vi "Simple TCP - Server.vi"() -> ()   [LabVIEW 2024]
doc: "Demonstrates how to set up a basic TCP connection, send data to the specified port once a connection has been established, and terminate the connection once the data has been sent. This VI is designed to stop if the TCP connection is terminated. The data sent in this example is an array of random numbers."
panel:
  in  "Client Closed":string="The client VI closed the connection."
  out "Waveform Graph":dbl[](graph)
  # "Overview: Demonstrates the use of the TCP functions to initialize a TCP server that can send data to a client VI.\nInstructions:\n1. Run the VI.\n2. Open Simple TCP - Client.vi and follow the instructions on its front panel. Note that if you wait longer than 30 seconds to do this after running this VI, it will time out.\n3. Click Stop on Simple TCP - Client.vi. This VI will stop automatically."
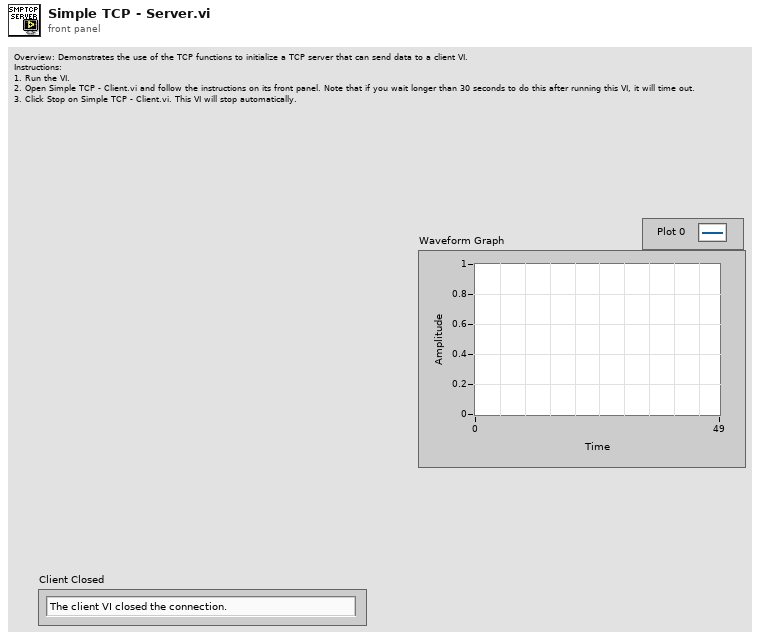
[diagram p1: front panel]
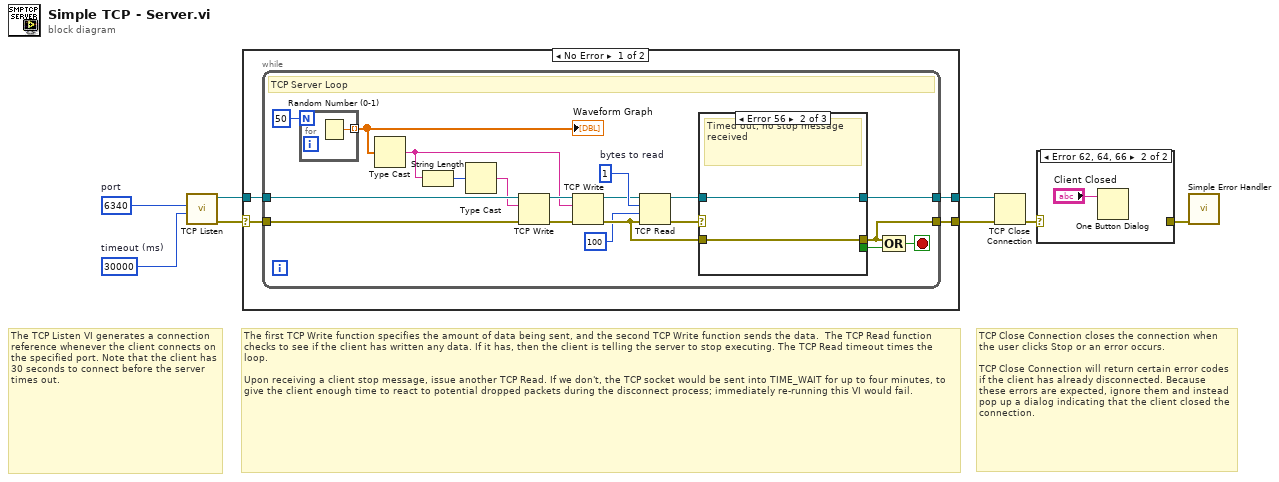
[diagram p0: block diagram]
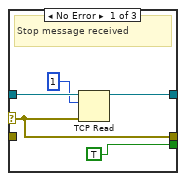
[diagram p2: hidden frame]
diagram:
  w3 = u16 6340  # port
  w4 = 30000  # timeout (ms)
  # "TCP Close Connection closes the connection when the user clicks Stop or an error occurs.\n\nTCP Close Connection will return certain error codes if the client has already disconnected. Because these errors are expected, ignore them and instead pop up a dialog indicating that the client closed the connection."
  # "The TCP Listen VI generates a connection reference whenever the client connects on the specified port. Note that the client has 30 seconds to connect before the server times out."
  # "The first TCP Write function specifies the amount of data being sent, and the second TCP Write function sends the data.  The TCP Read function checks to see if the client has written any data. If it has, then the client is telling the server to stop executing. The TCP Read timeout times the loop.\n\nUpon receiving a client stop message, issue another TCP Read. If we don't, the TCP socket would be sent into TIME_WAIT for up to four minutes, to give the client enough time to react to potential dropped packets during the disconnect process; immediately re-running this VI would fail."
  n1 = call <vilib>:"TCP Listen.vi"("timeout ms (wait forever: -1)"=w4, "port"=w3) -> ("error out"=w5:errorcluster, "connection ID"=w6:refnum<k5>)  [unwired: 5 in, 3 out]
  n2 = case shown="No Error" w5 {
    selector: w5 -> [w11 w43]
    tunnel: w6 -> [w12 w42]
    tunnel: [w10 w43] -> w2
    tunnel: [w9 w42] -> w1
    frame No Error {
      n3 = while {
        tunnel: [w19] -> w10
        tunnel: [w14] -> w9
        tunnel: w12 -> [w31]
        tunnel: w11 -> [w23]
        stop <- w25 stop-if-true
        w22 = 1  # bytes to read
        # "TCP Server Loop"
        n4 = for {
          N: 50 ("# of Points") -> [_]
          tunnel: [w41] -> w13 mode=indexing
          n5 = Random Number (0-1)() -> (number: 0 to 1=w41:dbl)
        }
        "Waveform Graph" <- w13
        n6 = Type Cast(x=w13) -> (*(type *) &x=w26:string)  [unwired: 1 out]
        n7 = String Length(string=w26) -> (length=w28:i32)
        n8 = Type Cast(x=w28) -> (*(type *) &x=w27:string)  [unwired: 1 out]
        n9 = TCP Write(connection ID=w31, data in=w27, error in (no error)=w23) -> (connection ID out=w30:refnum<k5>, error out=w29:errorcluster)  [unwired: 2 out]
        n10 = TCP Write(connection ID=w30, data in=w26, error in (no error)=w29) -> (connection ID out=w21:refnum<k5>, error out=w18:errorcluster)  [unwired: 2 out]
        n11 = TCP Read(connection ID=w21, bytes to read=w22, error in (no error)=w18, 9:100 ("milliseconds to wait")) -> (connection ID out=w15:refnum<k5>, error out=w20:errorcluster)  [unwired: 2 out]
        n12 = case shown="Error 56" w20 {
          selector: w20 -> [w33 _ w40]
          tunnel: [w33 w38 w40] -> w19
          tunnel: w18 -> [_ w38 _]
          tunnel: [TRUE _ _] -> w17
          tunnel: w15 -> [w35 w37 w39]
          tunnel: [w34 w37 w39] -> w14
          frame No Error {
            # "Stop message received"
            n13 = TCP Read(connection ID=w35, bytes to read=1, error in (no error)=w33) -> (connection ID out=w34:refnum<k5>)  [unwired: 1 in, 3 out]
          }
          frame Error {
            # "Timed out; no stop message received"
          }
          frame Default {
            # "Some other error occurred"
          }
        }
        n14 = Compound Arithmetic op=OR(w19, w17) -> (w25:bool)
      }
    }
    frame Error {
    }
  }
  n15 = TCP Close Connection(connection ID=w1, error in (no error)=w2) -> (error out=w8:errorcluster)  [unwired: 2 out]
  n16 = case shown="Error 62, 64, 66" w8 {
    selector: w8 -> [w44 _]
    tunnel: [w44 _] -> w7
    frame #0 {
    }
    frame #1 {
      n17 = One Button Dialog(message="Client Closed") -> ()  [unwired: 1 in, 1 out]
    }
  }
  n18 = call <vilib>:"Simple Error Handler.vi"("error in (no error)"=w7) -> ()  [unwired: 1 in, 8 out]
